vi "armControl.vi"(7 "Off":bool, 8 "locationPythonCode":path=path "C:/Users/ienoc/PycharmProjects/pythoXarmIanTest/starArmControl.py", 9 "pythonVersionIn":dbl=3.9, 10 "commandInput":string) -> (0 "armError":errorcluster, 1 "locationPythonCodeOutput":path=path "C:/Users/coralProgram/Documents/armand/xArm-Python-SDK-master/main.py", 2 "pythonVersionOut":dbl=3.9, 3 "pythonOutput":string)   [LabVIEW 2021]
panel:
  # "Inputs"
  # "Outputs"
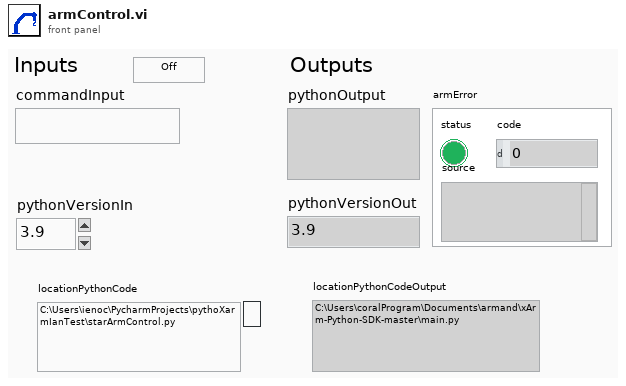
[diagram p1: front panel]
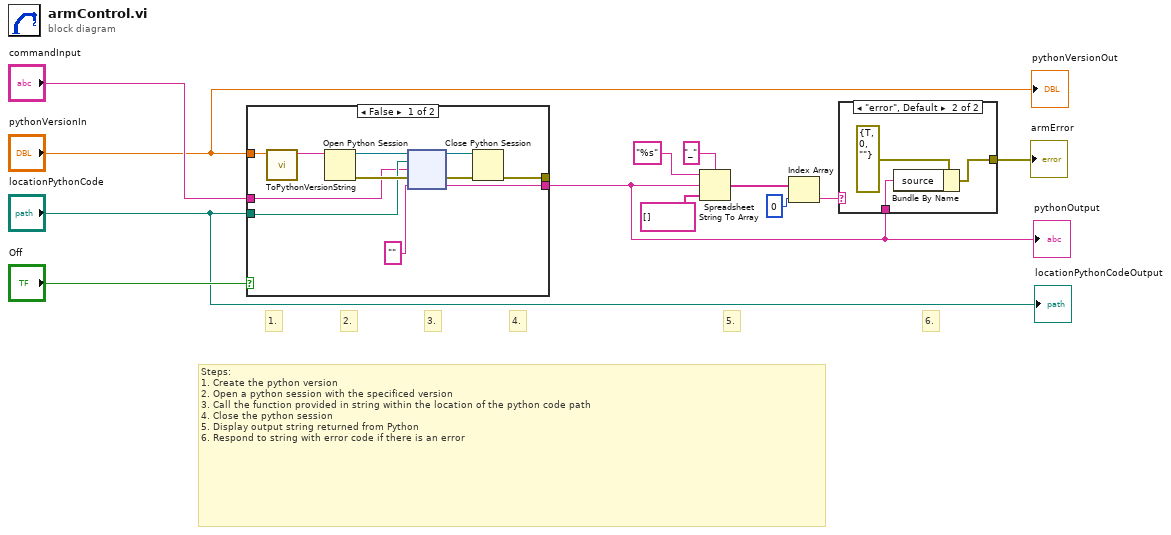
[diagram p0: block diagram]
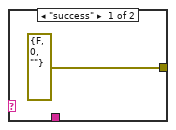
[diagram p2: hidden frame]
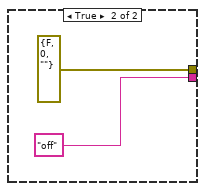
[diagram p3: hidden frame]
diagram:
  # "6."
  # "5."
  # "4."
  # "3."
  # "2."
  # "1."
  # "Steps:\n1. Create the python version\n2. Open a python session with the specificed version\n3. Call the function provided in string within the location of the python code path\n4. Close the python session\n5. Display output string returned from Python\n6. Respond to string with error code if there is an error"
  n1 = case shown="False" "Off" {
    tunnel: [w19 "off"] -> w1
    tunnel: [w16 errorcluster {"status"=FALSE, "code"=0, "source"=""} ("error out")] -> _
    tunnel: "pythonVersionIn" -> [w15 _]
    tunnel: "locationPythonCode" -> [w14 _]
    tunnel: "commandInput" -> [w13 _]
    frame False {
      n2 = call "ToPythonVersionString.vi"("python version"=w15) -> ("python version string"=w23:string)  [unwired: 10 in]
      n3 = Open Python Session(python version=w23) -> (session out=w22:refnum<k35>, error out=w18:errorcluster)  [unwired: 2 in]
      n4 = node(w22, w14, w13, w18, "" ("str1")) -> (w21:refnum<k35>, w17:errorcluster, w19:string)  [unwired: 2 out]
      n5 = Close Python Session(session in=w21, error in=w17) -> (11:w16:errorcluster)
    }
    frame True {
    }
  }
  "pythonOutput" <- w1
  n6 = Spreadsheet String To Array(delimiter (Tab)="_", format string="%s", spreadsheet string=w1, array type (2D Dbl)=string[] []) -> (array=w4:string[])
  n7 = Index Array(array=w4, index=0) -> (element=w2:string)
  n8 = case shown="\"error\", Default" w2 {
    tunnel: [errorcluster {"status"=FALSE, "code"=0, "source"=""} ("error out") w27] -> w11
    tunnel: w1 -> [_ w29]
    frame "success" {
    }
    frame "error", Default {
      n9 = Bundle By Name(cluster=errorcluster {"status"=TRUE, "code"=0, "source"=""} ("error out"), "source"=w29) -> (w27:errorcluster)
    }
  }
  "armError" <- w11
  "pythonVersionOut" <- "pythonVersionIn"
  "locationPythonCodeOutput" <- "locationPythonCode"
